vi "Teardown.vi"(8 "Error in":errorcluster, 9 "Teardown Location":T1, 10 "Unheard Msgs":refnum<class "Msg.lvclass">[](array[class]), 11 "TEMPLATE Actor in":refnum<class "TEMPLATE Actor.lvclass">) -> (3 "TEMPLATE Actor out":refnum<class "TEMPLATE Actor.lvclass">)   [LabVIEW 2020, in "_Template.lvlib" / "Templates.lvlib" / "TEMPLATE jettl Actor.lvlib" / "TEMPLATE Actor.lvlib" / "TEMPLATE Actor.lvclass"]
uses:
  TEMPLATE Actor.lvclass
  jettl/jettl/Msg/Msg.lvclass
  TEMPLATE Actor.lvclass/TEMPLATE Actor.ctl
  jettl/jettl/Actor/Actor.lvclass
  jettl/jettl/Teardown Location.ctl
  jettl/jettl/jettl.lvlib
panel:
  # "This front panel should not be manipulated."
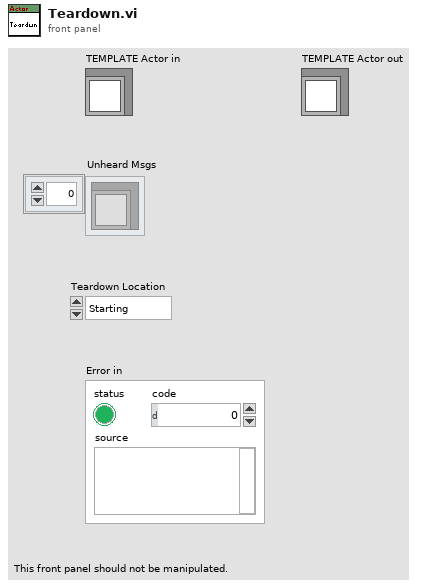
[diagram p1: front panel]
types:
  T1 = typedef "jettl.lvlib/Teardown Location.ctl" = enum16{"Starting", "Should Stop"}
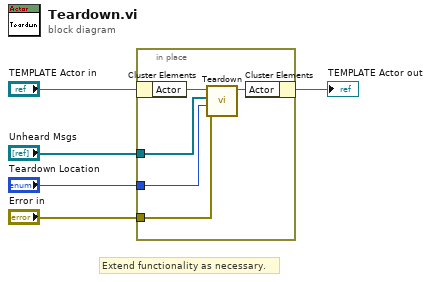
[diagram p0: block diagram]
diagram:
  # "Extend functionality as necessary."
  n1 = in-place {
    in-place-border: "Unheard Msgs" -> [w8]
    in-place-border: "Teardown Location" -> [w7]
    in-place-border: "Error in" -> [w6]
    n2 = in-place-cluster #1("TEMPLATE Actor in") -> ("Actor"=w10:refnum<class "Actor.lvclass">)
    n3 = call-dynamic "Teardown.vi"("Error in"=w6, "Teardown Location"=w7, "Unheard Msgs"=w8, "Actor in"=w10) -> ("Actor out"=w9:refnum<class "Actor.lvclass">)  [unwired: 7 in]
    n4 = in-place-cluster #1("Actor"=w9) -> (→"TEMPLATE Actor out":refnum<class "TEMPLATE Actor.lvclass">)
  }
